vi "LMS_self_design.vi"(9 "step_delta":cdb, 10 "train":cdb[](array[numeric]), 11 "sig":cdb[](array[numeric])) -> (1 "error":dbl[](array[numeric]), 2 "coe":cdb[](array[numeric]), 3 "filter_out":cdb[](array[numeric]))   [LabVIEW 2010]
panel:
  out "数值":i32
  in  "sig 2":dbl[](graph)
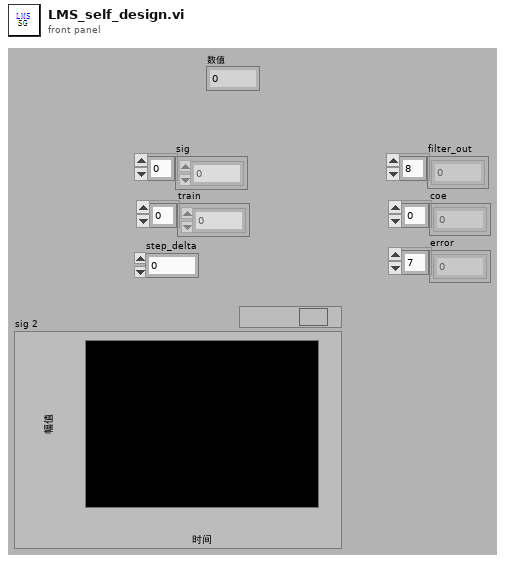
[diagram p1: front panel]
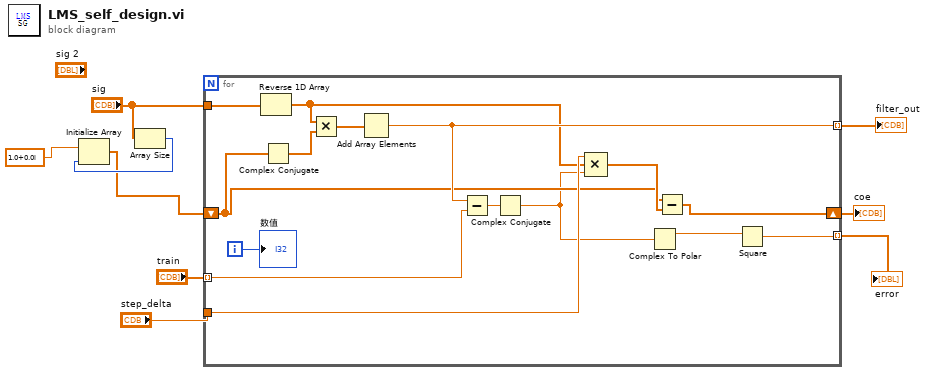
[diagram p0: block diagram]
diagram:
  n1 = Array Size(array="sig") -> (size(s)=w2:i32)
  n2 = Initialize Array(cdb 1.0+0.0i, w2) -> (w1:cdb[])
  n3 = for {
    shift-right: [w16] -> w6
    shift-left: w1 -> [w17]
    tunnel: [w22] -> w7 mode=indexing
    tunnel: [w13] -> w5 mode=indexing
    tunnel: "sig" -> [w12]
    tunnel: "train" -> [w11] mode=indexing
    tunnel: "step_delta" -> [w20]
    i -> [w10]
    n4 = Reverse 1D Array(array=w12) -> (reversed array=w19:cdb[])
    n5 = Complex Conjugate(1:w17) -> (0:w24:cdb[])
    n6 = Multiply(x=w19, y=w24) -> (x*y=w23:cdb[])
    n7 = Add Array Elements(numeric array=w23) -> (sum=w22:cdb)
    n8 = Subtract(x=w22, y=w11) -> (x-y=w21:cdb)
    n9 = Complex Conjugate(1:w21) -> (0:w15:cdb)
    n10 = Compound Arithmetic op=MULTIPLY(w20, w19, w15) -> (w18:cdb[])
    n11 = Complex To Polar(r * e^(i*theta)=w15) -> (r=w14:dbl)  [unwired: 1 out]
    n12 = Subtract(x=w17, y=w18) -> (x-y=w16:cdb[])
    n13 = Square(x=w14) -> (x^2=w13:dbl)
    "数值" <- w10
  }
  "filter_out" <- w7
  "coe" <- w6
  "error" <- w5
